vi "CreateBaseScripter.vi"(1 "Ctl Refnum":refnum<vi>, 2 "LVClassLibrary Ref":refnum<vi>) -> (0 "Scripter Out":refnum<class "BaseAccessorScripter.lvclass">)   [LabVIEW 2021, in "MemberVICreation.lvlib" / "BaseAccessorScripter.lvclass"]
uses:
  <resource>/Framework/Providers/LVClassLibrary/NewAccessors/BaseAccessorScripter/BaseAccessorScripter.lvclass
  <resource>/Framework/Providers/LVClassLibrary/NewAccessors/BaseAccessorScripter/BaseAccessorScripter.lvclass/BaseAccessorScripter.ctl
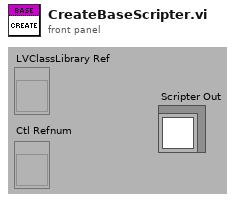
[diagram p1: front panel]
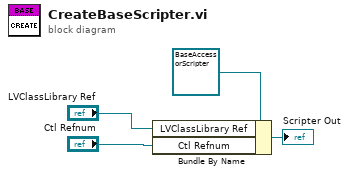
[diagram p0: block diagram]
diagram:
  n1 = Bundle By Name(cluster=refnum<class "BaseAccessorScripter.lvclass"> refnum ("AccessorCreation.lvlib:BaseAccessorScripter.lvclass"), "LVClassLibrary Ref"="LVClassLibrary Ref", "Ctl Refnum"="Ctl Refnum") -> (→"Scripter Out":refnum<class "BaseAccessorScripter.lvclass">)
